vi "NaN Trap.vi"(11 "Elevation in":dbl) -> (2 "NaN Detected":bool=TRUE, 3 "Elevation out":dbl)   [LabVIEW 2017]
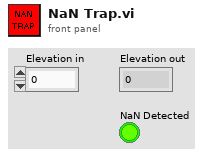
[diagram p1: front panel]
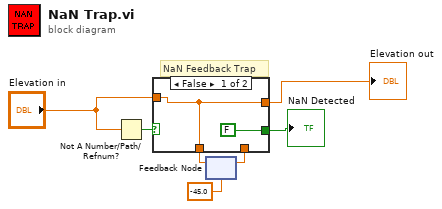
[diagram p0: block diagram]
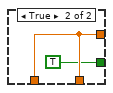
[diagram p2: hidden frame]
diagram:
  # "NaN Feedback Trap"
  n1 = Not A Number/Path/Refnum?(number/path/refnum="Elevation in") -> (NaN/Path/Refnum?=w5:bool)
  n2 = feedback #1(-45.0 ("Elevation")) -> (w2:dbl)
  n3 = case shown="False" w5 {
    tunnel: "Elevation in" -> [w9 _]
    tunnel: [w9 w11] -> w4
    tunnel: [w9 w11] -> w1
    tunnel: w2 -> [_ w11]
    tunnel: [FALSE ("Boolean") TRUE] -> w6
    frame False {
    }
    frame True {
    }
  }
  "NaN Detected" <- w6
  "Elevation out" <- w4
  n4 = feedback-in #1(w1) -> ()
